vi "FlattenShip.vi"(8 "error in":errorcluster, 9 "MainCluster _OUT":T9, 11 "Picture_IN":picture) -> (0 "error out":errorcluster, 3 "Picture_OUT":picture)   [LabVIEW 2019]
uses:
  InitCluster.ctl
  CharacterCluster.ctl
  <vilib>/picture/picture.llb/imagedata.ctl
  ShotInitCluster.ctl
  <vilib>/Utility/miscctls.llb/LVPositionTypeDef.ctl
  <vilib>/Utility/miscctls.llb/LVBoundsTypeDef.ctl
  InvaderPositionArray.ctl
  move_dir_lr.ctl
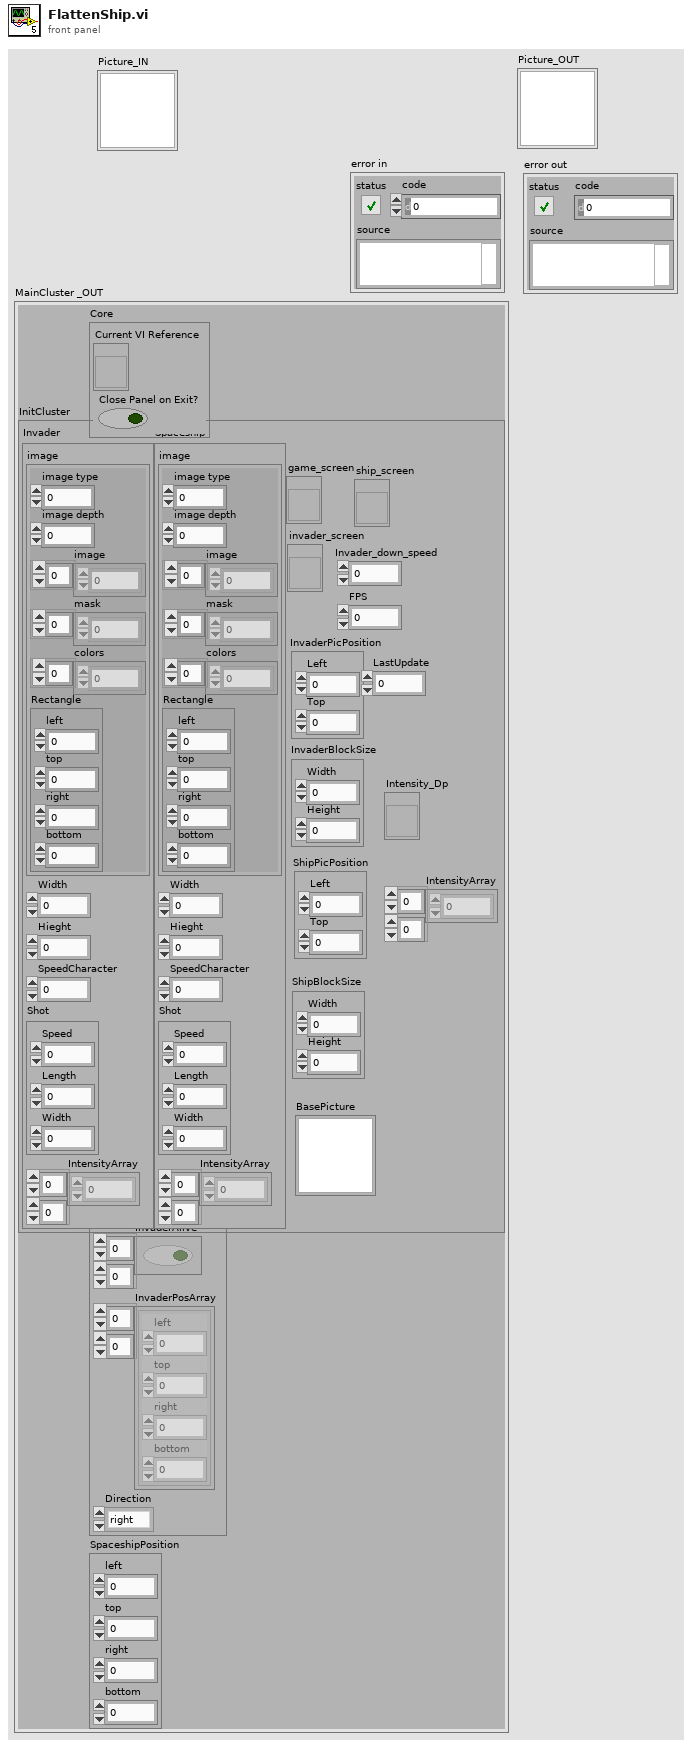
[diagram p1: front panel]
types:
  T1 = typedef "InitCluster.ctl" = cluster{"Invader":T2, "Spaceship":T2, "game_screen":refnum<vi>, "BasePicture":picture, "invader_screen":refnum<vi>, "InvaderPicPosition":T5, "Invader_down_speed":i16, "FPS":u16, "InvaderBlockSize":T6, "ship_screen":refnum<vi>, "ShipBlockSize":T6, "ShipPicPosition":T5, "LastUpdate":u32, "Intensity_Dp":refnum<vi>, "IntensityArray":u8[][]}
  T2 = typedef "CharacterCluster.ctl" = cluster{"image":T3, "Width":u32, "Hieght":u32, "SpeedCharacter":u32, "Shot":T4, "IntensityArray":u8[][]}
  T3 = typedef "imagedata.ctl" = cluster{"image type":i32, "image depth":i32, "image":u8[], "mask":u8[], "colors":u32[], "Rectangle":cluster{"left":i16, "top":i16, "right":i16, "bottom":i16}}
  T4 = typedef "ShotInitCluster.ctl" = cluster{"Speed":u32, "Length":u32, "Width":u32}
  T5 = typedef "LVPositionTypeDef.ctl" = cluster{"Left":i32, "Top":i32}
  T6 = typedef "LVBoundsTypeDef.ctl" = cluster{"Width":u32, "Height":u32}
  T7 = typedef "InvaderPositionArray.ctl" = cluster{"InvaderAlive":bool[][], "InvaderPosArray":cluster{"left":i16, "top":i16, "right":i16, "bottom":i16}[][], "Direction":T8}
  T8 = typedef "move_dir_lr.ctl" = enum16{"right", "left"}
  T9 = cluster{"Core":cluster{"Current VI Reference":refnum<vi>, "Close Panel on Exit?":bool}, "InitCluster":T1, "InvaderPosArray":T7, "SpaceshipPosition":cluster{"left":i16, "top":i16, "right":i16, "bottom":i16}}
  T10 = cluster{"left":i16, "top":i16, "right":i16, "bottom":i16}
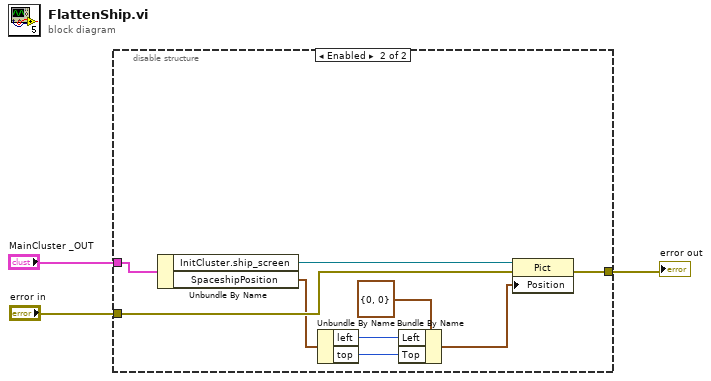
[diagram p0: block diagram]
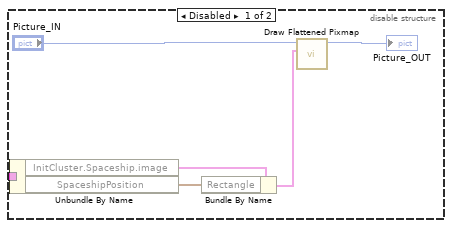
[diagram p2: hidden frame]
diagram:
  n1 = disable-structure shown="Enabled" {
    disable-tunnel: "MainCluster _OUT" -> [w7 w18]
    disable-tunnel: "error in" -> [_ w16]
    disable-tunnel: [_ w10] -> w1
    frame Disabled {
      n2 = Unbundle By Name(w7) -> ("InitCluster.Spaceship.image"=w6:T3, "SpaceshipPosition"=w5:T10)
      n3 = Bundle By Name(cluster=w6, "Rectangle"=w5) -> (w4:T3)
      n4 = call <vilib>:"Draw Flattened Pixmap.vi"("image data"=w4, "picture"="Picture_IN") -> ("new picture"=→"Picture_OUT":picture)  [unwired: 7 in]
    }
    frame Enabled {
      n5 = Unbundle By Name(w18) -> ("InitCluster.ship_screen"=w17:refnum<vi>, "SpaceshipPosition"=w15:T10)
      n6 = Unbundle By Name(w15) -> ("left"=w13:i16, "top"=w12:i16)
      n7 = Bundle By Name(cluster=T5 {"Left"=0, "Top"=0} ("Position"), "Left"=w13, "Top"=w12) -> (w11:T5)
      n8 = property class="Pict"(reference=w17, error in=w16, "Position"=w11) -> (error out=w10:errorcluster)  [unwired: 1 out]
    }
  }
  "error out" <- w1
